vi "Display_LDA_data_rate.vi"(1 "Hydrosonic Setting %":dbl, 2 "Current Sampling Freq (Hz)":dbl format="%#.0f") -> ()   [LabVIEW 2012]
panel:
  out "XY Graph":cluster{timestamp[], dbl[]}[](graph)
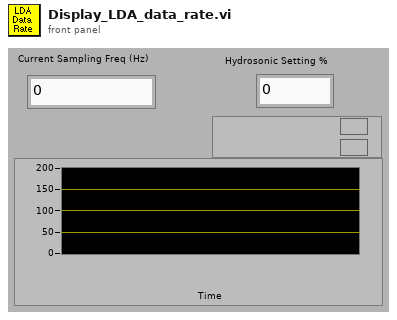
[diagram p1: front panel]
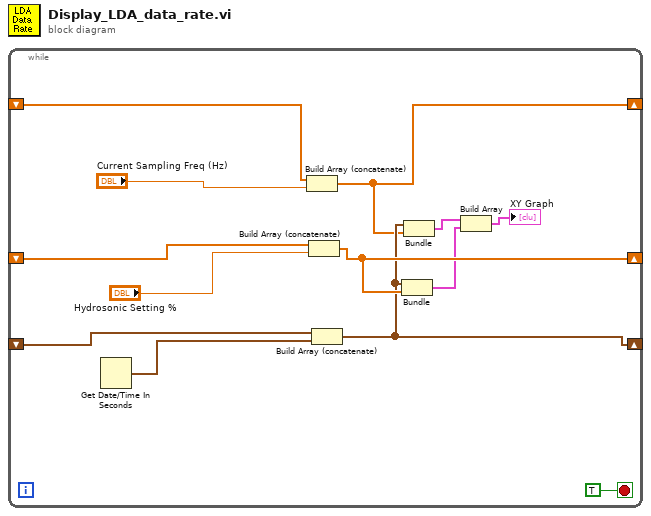
[diagram p0: block diagram]
diagram:
  n1 = while {
    shift-right: [w5] -> _
    shift-left: _ -> [w12]
    shift-right: [w7] -> _
    shift-left: _ -> [w10]
    shift-right: [w6] -> _
    shift-left: _ -> [w8]
    stop <- TRUE stop-if-true
    n2 = Get Date/Time In Seconds() -> (seconds since 1Jan1904=w9:timestamp)
    n3 = Build Array (concatenate)(w12, "Current Sampling Freq (Hz)") -> (w5:dbl[])
    n4 = Build Array (concatenate)(w10, "Hydrosonic Setting %") -> (w7:dbl[])
    n5 = Build Array (concatenate)(w8, w9) -> (w6:timestamp[])
    n6 = Bundle(w6, w7) -> (w3:cluster{timestamp[], dbl[]})  [unwired: 1 in]
    n7 = Bundle(w6, w5) -> (w4:cluster{timestamp[], dbl[]})  [unwired: 1 in]
    n8 = Build Array(w4, w3) -> (→"XY Graph":cluster{timestamp[], dbl[]}[])
  }
